vi "Get Member VIs.vi"(8 "error in (no error)":errorcluster, 10 "Test Class Path":path) -> (0 "error out":errorcluster, 2 "Array":path[](array[path]))   [LabVIEW 2020, in "Pure Mock Class Generator Test.lvclass"]
uses:
  Pure Mock Class Generator Test.lvclass
  Pure Mock Class Generator Test.lvclass/Pure Mock Class Generator Test.ctl
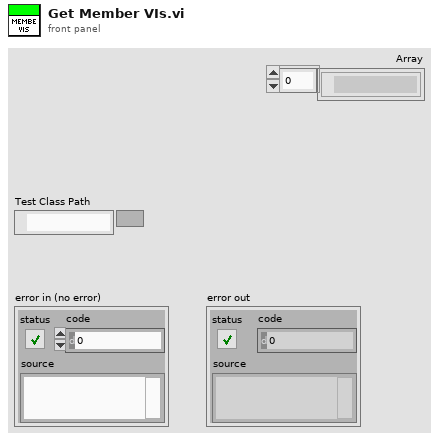
[diagram p1: front panel]
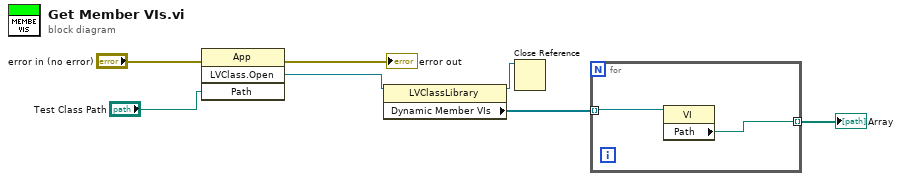
[diagram p0: block diagram]
diagram:
  n1 = invoke class="App" method="LVClass.Open"(error in="error in (no error)", "Path"="Test Class Path") -> (error out=→"error out":errorcluster, "LVClass.Open"=w4:refnum<vi>)  [unwired: 2 in, 2 out]
  n2 = property class="LVClassLibrary"(reference=w4) -> (reference out=w3:refnum<vi>, "Dynamic Member VIs"=w2:refnum<vi>[])  [unwired: 1 in, 1 out]
  n3 = Close Reference(reference=w3) -> ()  [unwired: 1 in, 1 out]
  n4 = for {
    tunnel: w2 -> [w9] mode=indexing
    tunnel: [w8] -> w1 mode=indexing
    n5 = property class="VI"(reference=w9) -> ("Path"=w8:path)  [unwired: 1 in, 2 out]
  }
  "Array" <- w1
